vi "Assert Equal Type_Variant.vi"(4 "Execution time (s)":dbl=-1.0, 6 "error code (1)":i32=1, 7 "Label":string, 8 "error in":errorcluster, 10 "Y":variant, 11 "X":variant) -> (0 "error out":errorcluster, 2 "Properties":refnum<class "Properties.Assert.lvclass">)   [LabVIEW 2021, in "Bananas.lvlib"]
uses:
  Bananas.lvlib
  <vilib>/addons/_JKI Toolkits/Caraya/classes/Assert/Assert.lvclass
  Banana/Banana.lvclass
  AssertEqualType/AssertEqualType.lvclass
  C:/Repositories/LVOS/Bananas/lv-src/Bananas/AssertEqualType/AssertEqualType.lvclass
  C:/Repositories/LVOS/Bananas/lv-src/Bananas/BananaPeel/BananaPeel.lvclass
  <vilib>/addons/_JKI Toolkits/Caraya/classes/Properties.Assert/Properties.Assert.lvclass
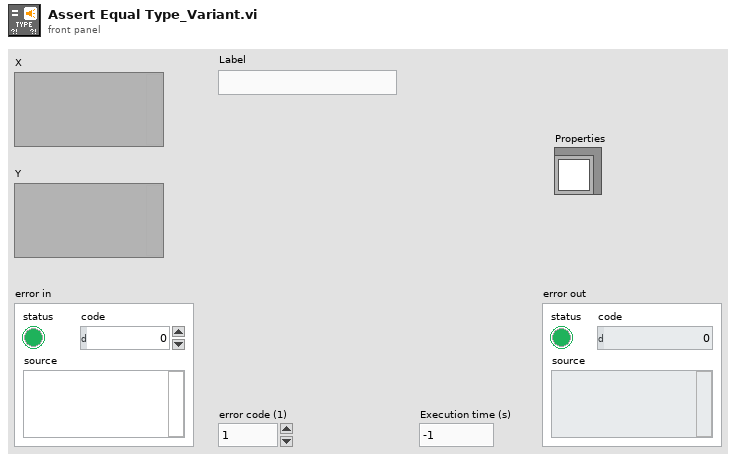
[diagram p1: front panel]
types:
  T1 = typedef "Bananas.lvlib/Assertion Strategies -- cluster.ctl" = cluster{"AssertTrue":refnum<class "AssertTrue.lvclass">, "AssertFalse":refnum<class "AssertFalse.lvclass">, "AssertEqualValue":refnum<class "AssertEqualValue.lvclass">, "AssertEqualType":refnum<class "AssertEqualType.lvclass">, "AssertCompareValue":refnum<class "AssertCompareValue.lvclass">, "AssertError":refnum<class "AssertError.lvclass">, "AssertAlmostEqual":refnum<class "AssertAlmostEqualValue.lvclass">}
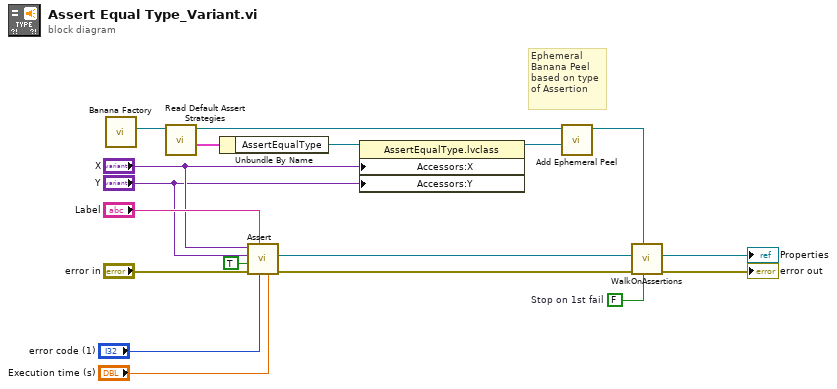
[diagram p0: block diagram]
diagram:
  w1 = FALSE  # Stop on 1st fail
  # "Ephemeral\nBanana Peel\nbased on type\nof Assertion"
  n1 = call "Banana Factory.vi"() -> ("Bunch"=w8:refnum<class "Banana.lvclass">)  [unwired: 10 in, 1 out]
  n2 = call "Read Default Assert Strategies.vi"("Banana in"=w8) -> ("Strategies"=w6:T1, "Banana out"=w7:refnum<class "Banana.lvclass">)  [unwired: 9 in]
  n3 = Unbundle By Name(w6) -> ("AssertEqualType"=w3:refnum<class "AssertEqualType.lvclass">)
  n4 = call-poly <vilib>:"Assert.vi"("Execution time (s)"="Execution time (s)", "error code (1)"="error code (1)", "Label"="Label", "error in (no error)"="error in", "Register with caller test (F)"=TRUE, "Y"="Y", "X"="X") -> ("error out"=w13:errorcluster, "Properties.Assert"=w11:refnum<class "Properties.Assert.lvclass">)  [unwired: 3 in]
  n5 = property class="AssertEqualType.lvclass"(reference=w3, "Accessors:X"="X", "Accessors:Y"="Y") -> (reference out=w2:refnum<class "AssertEqualType.lvclass">)  [unwired: 1 in, 1 out]
  n6 = call "Add Ephemeral Peel.vi"("BananaPeel"=w2, "Bunch"=w7) -> ("Bunch"=w9:refnum<class "Banana.lvclass">)  [unwired: 9 in]
  n7 = call "WalkOnAssertions.vi"("Stop on 1st fail"=w1, "Bunch"=w9, "error in (no error)"=w13, "Properties"=w11) -> ("error out"=→"error out":errorcluster, "Properties out"=→"Properties":refnum<class "Properties.Assert.lvclass">)  [unwired: 6 in]
